vi "ep_Read Type of Reference Voltage.vi"(8 "error in (no error)":errorcluster, 11 "system info in":refnum<class "EP System Info.lvclass">) -> (0 "error out":errorcluster, 2 "type of reference voltage":enum16{"Constant", "Sliding"}(ring), 3 "system info out":refnum<class "EP System Info.lvclass">)   [LabVIEW 2011, in "NI_EP_Power Quality.lvlib" / "EP System Info.lvclass"]
uses:
  <vilib>/addons/Electrical Power/PQ/Common/Classes/System Info/EP System Info.lvclass
  <vilib>/addons/Electrical Power/PQ/Common/Classes/System Info/EP System Info.lvclass/EP System Info.ctl
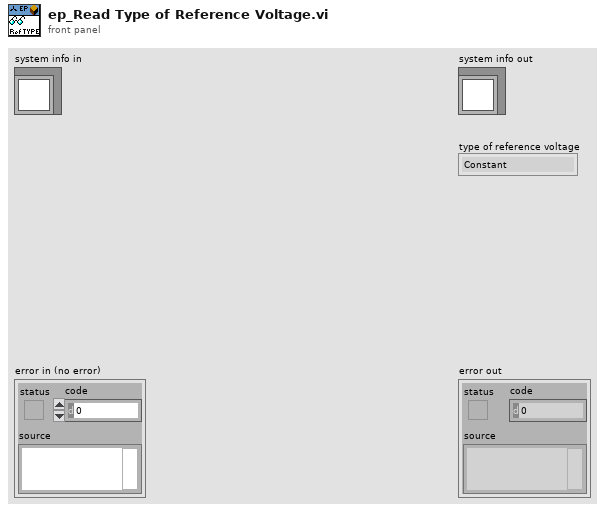
[diagram p1: front panel]
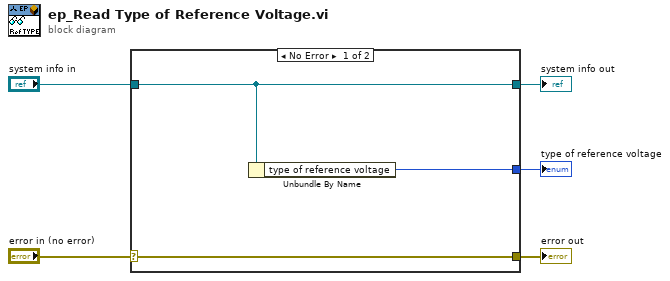
[diagram p0: block diagram]
diagram:
  n1 = case shown="No Error" "error in (no error)" {
    selector: "error in (no error)" -> [w8 w9]
    tunnel: [w8 w9] -> w4
    tunnel: [w6 w10] -> w2
    tunnel: "system info in" -> [w6 w10]
    tunnel: [w7 _] -> w1
    frame No Error {
      n2 = Unbundle By Name(w6) -> ("type of reference voltage"=w7:enum16{"Constant", "Sliding"})
    }
    frame Error {
    }
  }
  "error out" <- w4
  "system info out" <- w2
  "type of reference voltage" <- w1
